vi "OnDoubleClick.vi"(0 "XRef":T11, 1 "Point":T9, 2 "Mouse Mods":T7, 3 "State In":T1) -> (14 "Reply":T5, 15 "Fatal Error Out":T4, 16 "State Out":T1)   [LabVIEW 2018, in "RetryNode.xnode"]
uses:
  RetryNode.xnode
  <vilib>/XNodeSupport/XNodeXNodeRef.ctl
  <vilib>/XNodeSupport/XNodePoint.ctl
  <vilib>/XNodeSupport/XNodeInt.ctl
  <vilib>/XNodeSupport/XNodeMouseMods.ctl
  <vilib>/XNodeSupport/XNodeBool.ctl
  State.ctl
  <vilib>/Utility/miscctls.llb/LVRectTypeDef.ctl
  Options.ctl
  <vilib>/XNodeSupport/XNodeStringArray.ctl
  <vilib>/XNodeSupport/XNodeString.ctl
  <vilib>/XNodeSupport/XNodeErrorCluster.ctl
  <vilib>/XNodeSupport/NI_XNodeSupport.lvlib
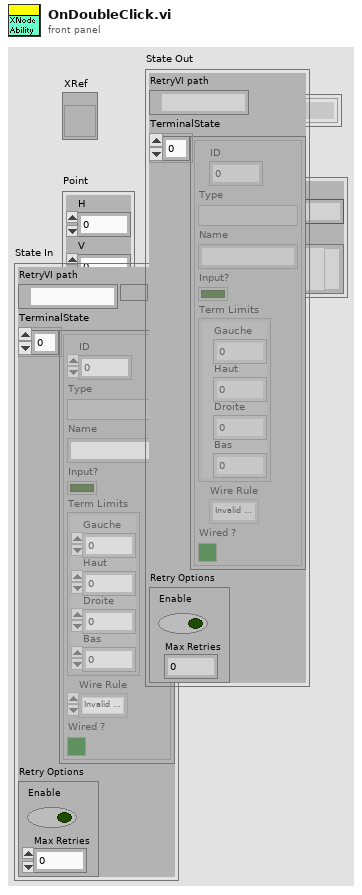
[diagram p1: front panel]
types:
  T1 = typedef "RetryNode.xnode/State.ctl" = cluster{"RetryVI path":path, "TerminalState":cluster{"ID":i32, "Type":variant, "Name":string, "Input?":bool, "Term Limits":T2, "Wire Rule":enum16{"Invalid Wire Rule", "Required", "Recommended", "Optional", "Dynamic Dispatch"}, "Wired ?":bool}[], "Retry Options":T3}
  T2 = typedef "LVRectTypeDef.ctl" = cluster{"Left":i16, "Top":i16, "Right":i16, "Bottom":i16}
  T3 = typedef "RetryNode.xnode/Options.ctl" = cluster{"Enable":bool, "Max Retries":i32}
  T4 = typedef "NI_XNodeSupport.lvlib/XNodeErrorCluster.ctl" = errorcluster
  T5 = typedef "NI_XNodeSupport.lvlib/XNodeStringArray.ctl" = T6[]
  T6 = typedef "NI_XNodeSupport.lvlib/XNodeString.ctl" = string
  T7 = typedef "NI_XNodeSupport.lvlib/XNodeMouseMods.ctl" = cluster{"Shift?":T8, "Menu?":T8, "Alt?":T8}
  T8 = typedef "NI_XNodeSupport.lvlib/XNodeBool.ctl" = bool
  T9 = typedef "NI_XNodeSupport.lvlib/XNodePoint.ctl" = cluster{"H":T10, "V":T10}
  T10 = typedef "NI_XNodeSupport.lvlib/XNodeInt.ctl" = i32
  T11 = typedef "NI_XNodeSupport.lvlib/XNodeXNodeRef.ctl" = refnum<vi>
  T12 = enum32{"Invalid", "Standard", "Closed", "Hidden", "Minimized", "Maximized"}
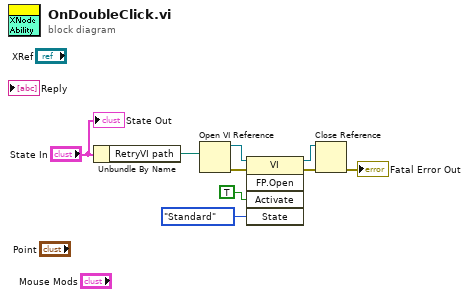
[diagram p0: block diagram]
diagram:
  n1 = Unbundle By Name("State In") -> ("RetryVI path"=w8:path)
  n2 = Open VI Reference(vi path=w8) -> (vi reference=w7:refnum<vi>, error out=w1:errorcluster)  [unwired: 5 in]
  n3 = invoke class="VI" method="FP.Open"(reference=w7, error in=w1, "Activate"=TRUE ("Activate?"), "State"=T12."Standard") -> (reference out=w3:refnum<vi>, error out=w4:errorcluster)  [unwired: 1 in, 3 out]
  n4 = Close Reference(reference=w3, error in (no error)=w4) -> (error out=→"Fatal Error Out":errorcluster)
  "State Out" <- "State In"
